vi "HAL camera get temp.vi"(0 "Cooling status In":T1) -> (1 "Error?":bool, 2 "Cooling status Out":T1, 3 "Current temperature":i32)   [LabVIEW 2011]
uses:
  HAL cooling status.ctt
  Cascade-specific globals.vi
panel:
  out "Setpoint from camera":dbl caption="Value" format="%.2f"
  in  "error in (no error)":errorcluster caption="error in"
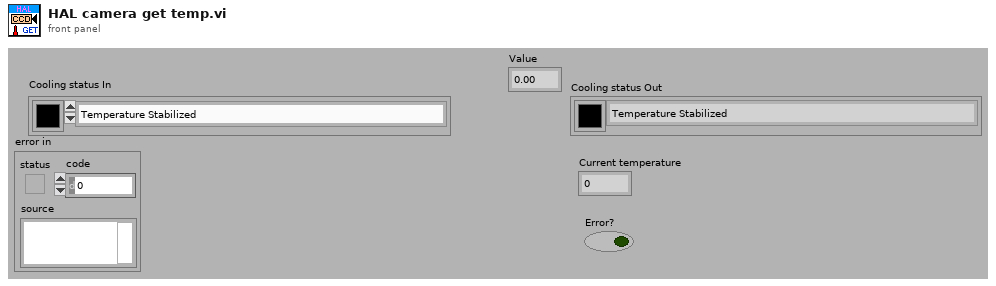
[diagram p1: front panel]
types:
  T1 = typedef "HAL cooling status.ctt" = cluster{"Color Box":u32, "Cooling Status":enum16{"Temperature Stabilized", "Waiting to Stabilize Temperature", "Cooling is Turned Off", "Have not yet Reached Set Temperature"}}
  T2 = enum16{"Temperature Stabilized", "Waiting to Stabilize Temperature", "Cooling is Turned Off"}
  T3 = enum16{"Temperature Stabilized", "Waiting to Stabilize Temperature", "Cooling is Turned Off", "Have not yet Reached Set Temperature"}
  T4 = cluster{"Camera Handle":u32, "Pulser Handle":u32, "File Handle":u32, "Display Handle":u32, "Image Handle":u32}
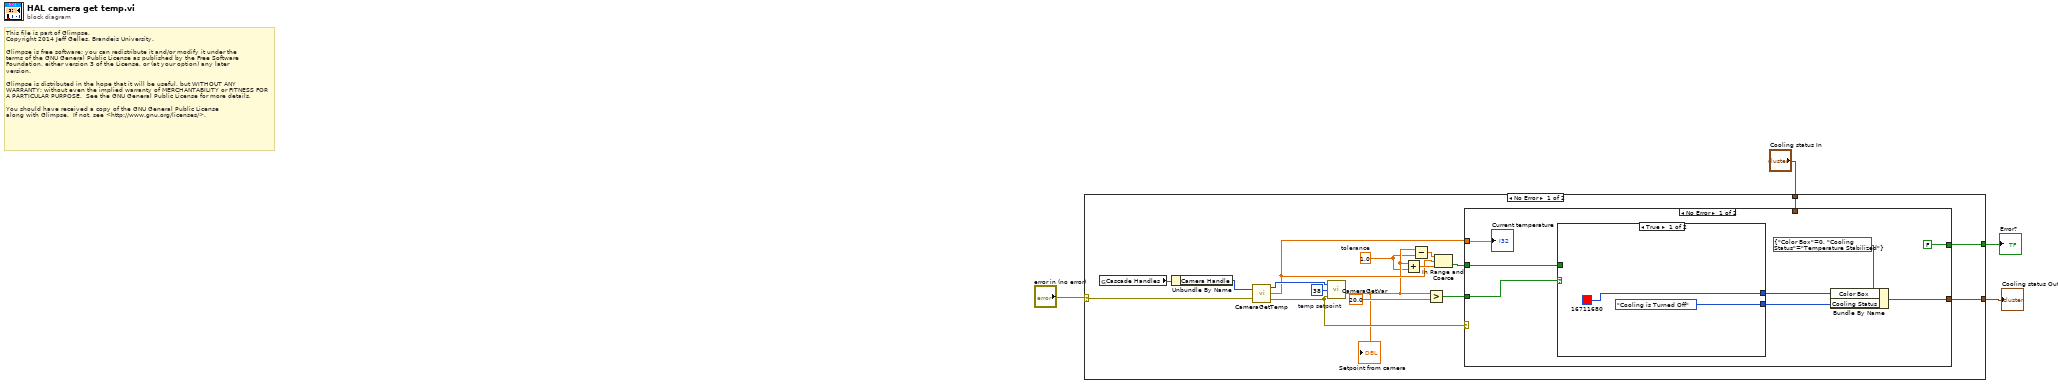
[diagram p0: block diagram]
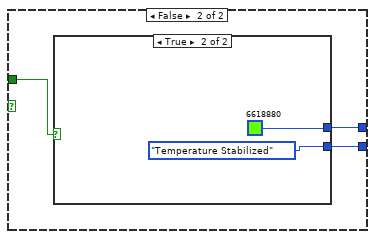
[diagram p2: hidden frame]
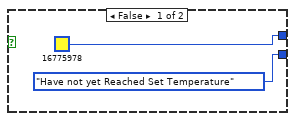
[diagram p3: hidden frame]
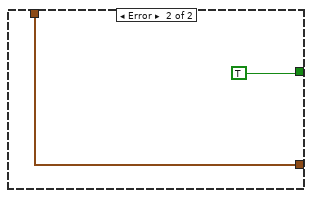
[diagram p4: hidden frame]
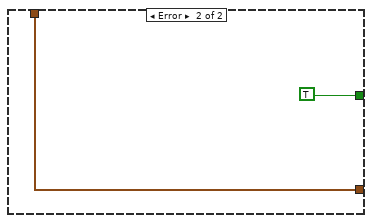
[diagram p5: hidden frame]
diagram:
  # "This file is part of Glimpse. \nCopyright 2014 Jeff Gelles, Brandeis University.    \n\nGlimpse is free software: you can redistribute it and/or modify it under the \nterms of the GNU General Public License as published by the Free Software \nFoundation, either version 3 of the License, or (at your option) any later \nversion.\n\nGlimpse is distributed in the hope that it will be useful, but WITHOUT ANY \nWARRANTY; without even the implied warranty of MERCHANTABILITY or FITNESS FOR \nA PARTICULAR PURPOSE.  See the GNU General Public License for more details.\n\nYou should have received a copy of the GNU General Public License\nalong with Glimpse.  If not, see <http://www.gnu.org/licenses/>."
  n1 = case shown="No Error" "error in (no error)" {
    selector: "error in (no error)" -> [w18 _]
    tunnel: [w9 w42] -> w3
    tunnel: [w8 TRUE ("Error?")] -> w2
    tunnel: "Cooling status In" -> [w7 w42]
    frame No Error {
      w11 = 1.0  # tolerance
      w21 = u32 38  # temp setpoint
      n2 = global read "Cascade-specific globals.vi" "Cascade Handles"() -> (w6:T4)
      n3 = Unbundle By Name(w6) -> ("Camera Handle"=w5:u32)
      n4 = call <userlib>:"CameraGetTemp.vi"("Camera Handle"=w5, "error in (no error)"=w18) -> ("Camera Handle"=w20:u32, "Temperature"=w13:dbl, "error out"=w17:errorcluster)
      n5 = call <userlib>:"CameraGetVar.vi"("error in"=w17, "Parameter ID"=w21, "Camera Handle"=w20) -> ("Value"=w12:dbl)  [unwired: 2 out]
      "Setpoint from camera" <- w12
      n6 = Add(x=w12, y=w11) -> (x+y=w15:dbl)
      n7 = Subtract(x=w12, y=w11) -> (x-y=w14:dbl)
      n8 = Greater?(x=w12, y=20.0) -> (0:w16:bool)
      n9 = In Range and Coerce(upper limit=w14, x=w13, lower limit=w15) -> (In Range?=w10:bool)  [unwired: 1 out]
      n10 = case shown="No Error" w17 {
        tunnel: w13 -> [w29 _]
        tunnel: w16 -> [w28 _]
        tunnel: w10 -> [w27 _]
        tunnel: [w23 w39] -> w9
        tunnel: [FALSE ("Error?") TRUE ("Error?")] -> w8
        tunnel: w7 -> [_ w39]
        frame No Error {
          n11 = case shown="True" w28 {
            tunnel: [u32 16711680 w33] -> w25
            tunnel: [T2."Cooling is Turned Off" ("Cooling Status") w32] -> w24
            tunnel: w27 -> [_ w34]
            frame True {
            }
            frame False {
              n12 = case shown="True" w34 {
                tunnel: [u32 16775978 u32 6618880] -> w33
                tunnel: [T3."Have not yet Reached Set Temperature" ("Cooling Status") T2."Temperature Stabilized" ("Cooling Status")] -> w32
                frame False {
                }
                frame True {
                }
              }
            }
          }
          n13 = Bundle By Name(cluster=T1 {"Color Box"=0, "Cooling Status"=enum."Temperature Stabilized"} ("Cooling status"), "Color Box"=w25, "Cooling Status"=w24) -> (w23:T1)
          "Current temperature" <- w29
        }
        frame Error {
        }
      }
    }
    frame Error {
    }
  }
  "Error?" <- w2
  "Cooling status Out" <- w3
